vi "Nelson_Whale_Tracker.vi"() -> ()   [LabVIEW 2014]
uses:
  <vilib>/userdefined/High Color/IMAQdx.ctl
  <vilib>/vision/driver/IMAQdx.llb/IMAQdx Attribute Type.ctl
  <vilib>/vision/driver/NI_Vision_Acquisition_Software.lvlib
  <resource>/objmgr/imaqdx.rc
panel:
  in  "Tab Control":enum32{"Whale Tracker", "Diagnostics"}(tab)
  in  "Color Based\nTracking?":bool=TRUE
  out "Image":T1(plugin-control)
  in  "Session In":T2="cam1"
  in  "Image Type":T3=4 items=["Grayscale (U8)", "Grayscale (I16)", "Grayscale (SGL)", "Complex (CSG)", "RGB (U32)", "HSL (U32)", "RGB (U64)", "Grayscale (U16)"]
  out "Whale Position":cluster{"Y":dbl, "X":dbl}
  out "Crosshairs Display":T1(plugin-control)
  in  "Crosshairs Image Type":T3=1 items=["Grayscale (U8)", "Grayscale (I16)", "Grayscale (SGL)", "Complex (CSG)", "RGB (U32)", "HSL (U32)", "RGB (U64)", "Grayscale (U16)"]
  in  "Crosshairs Path":path=path "C:/Users/dnelson1/Desktop/Work/!Classes/Robo I/VISION/2014 Source Images/Crosshairs_Small.bmp"
  out "error out":errorcluster
  out "Attribute Information Array":T5(array[cluster])
  out "Attribute Name":string
  in  "Stop":bool
  out "Running":bool
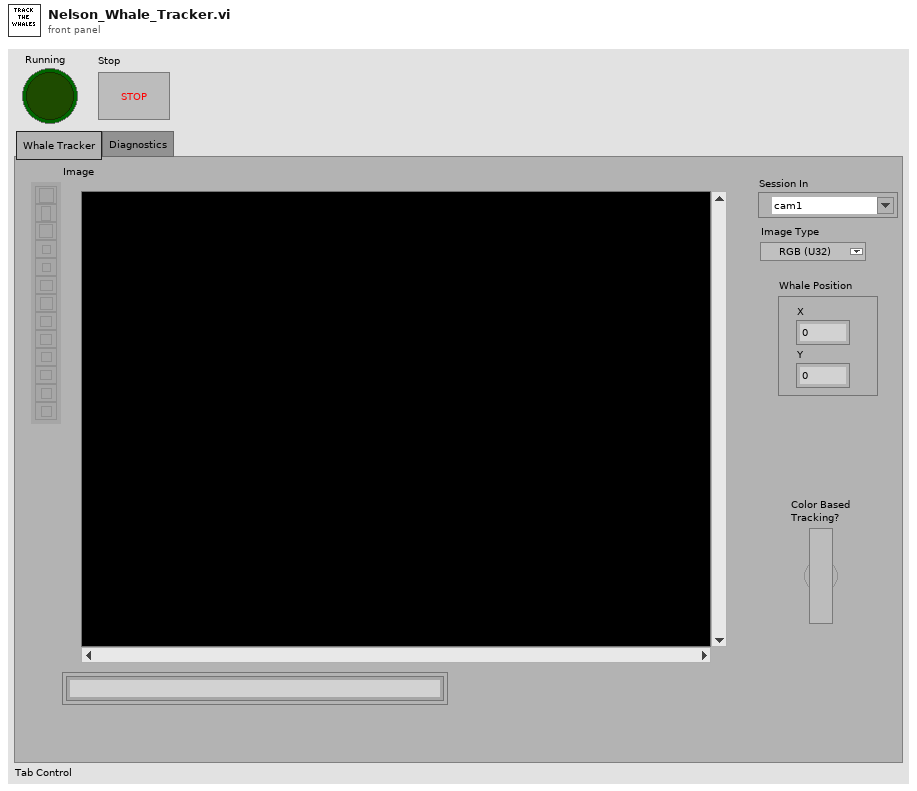
[diagram p1: front panel]
types:
  T1 = typedef "IMAQ Image.ctl" = refnum<image>
  T2 = typedef "IMAQdx.ctl" = refnum<k21>
  T3 = typedef "Image Type" = u32
  T4 = typedef "NI_Vision_Acquisition_Software.lvlib/IMAQdx Attribute Type.ctl" = enum32{"U32", "I64", "DBL", "String", "Enum", "Bool", "Command"}
  T5 = cluster{"Attribute Type":T4, "Readable":bool, "Writable":bool, "Attribute Name":string}[]
  T6 = cluster{"Attribute Type":T4, "Readable":bool, "Writable":bool, "Attribute Name":string}
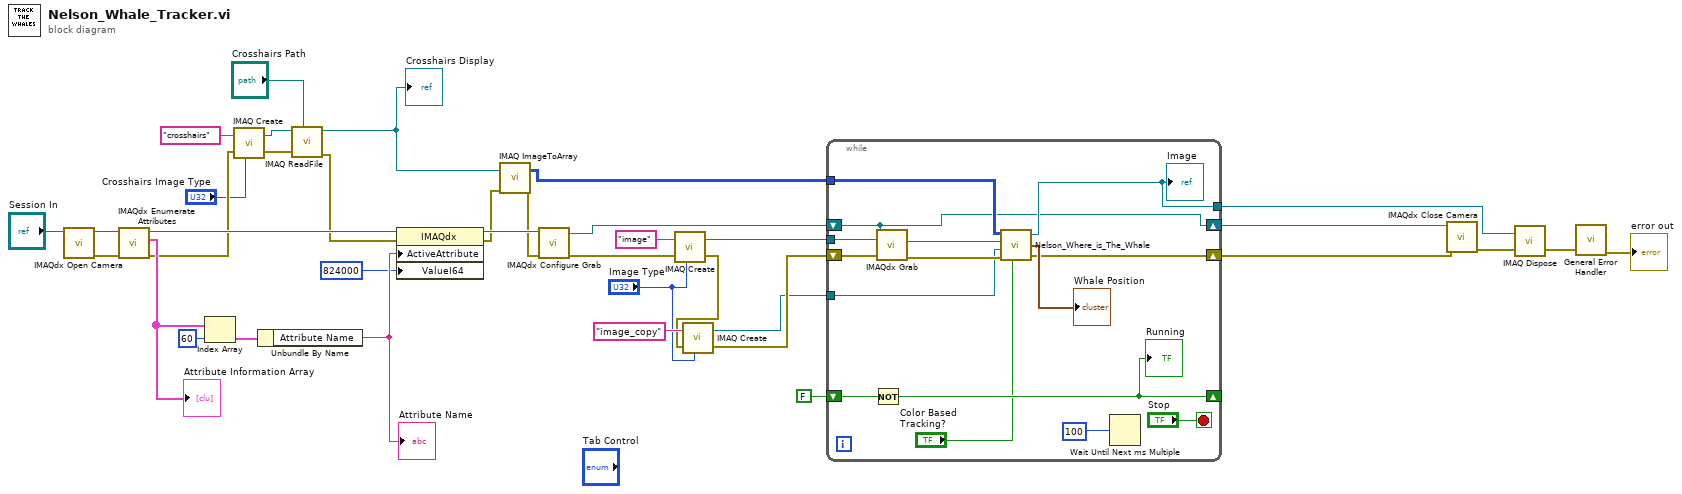
[diagram p0: block diagram]
diagram:
  n1 = call <vilib>:"IMAQdx Open Camera.vi"("Session In"="Session In") -> ("error out"=w35:errorcluster, "Session Out"=w36:T2)  [unwired: 9 in]
  n2 = call <vilib>:"IMAQdx Enumerate Attributes.vi"("error in"=w35, "Session In"=w36) -> ("error out"=w16:errorcluster, "Attribute Information Array"=w32:T5, "Session Out"=w34:T2)  [unwired: 7 in]
  "Attribute Information Array" <- w32
  n3 = Index Array(array=w32, index=60) -> (element=w31:T6)
  n4 = call "IMAQ Create"("Image Name"="crosshairs", "Image Type"="Crosshairs Image Type", "error in (no error)"=w16) -> ("New Image"=w18:T1, "error out"=w17:errorcluster)  [unwired: 2 in]
  n5 = Unbundle By Name(w31) -> ("Attribute Name"=w30:string)
  "Attribute Name" <- w30
  n6 = call "IMAQ ReadFile"("File Path"="Crosshairs Path", "error in (no error)"=w17, "Image"=w18) -> ("error out"=w14:errorcluster, "Image Out"=w10:T1)  [unwired: 4 in, 3 out]
  "Crosshairs Display" <- w10
  n7 = property class="IMAQdx"(reference=w34, error in=w14, "ActiveAttribute"=w30, "ValueI64"=i64 824000) -> (reference out=w28:T2, error out=w2:errorcluster)
  n8 = call "IMAQ ImageToArray"("error in (no error)"=w2, "Image"=w10) -> ("error out"=w1:errorcluster, "Image Pixels (I16)"=w11:i16[][])  [unwired: 2 in, 3 out]
  n9 = call <vilib>:"IMAQdx Configure Grab.vi"("error in"=w1, "Session In"=w28) -> ("error out"=w27:errorcluster, "Session Out"=w24:T2)  [unwired: 8 in]
  n10 = call "IMAQ Create"("Image Name"="image", "Image Type"="Image Type", "error in (no error)"=w27) -> ("New Image"=w25:T1, "error out"=w7:errorcluster)  [unwired: 2 in]
  n11 = call "IMAQ Create"("Image Name"="image_copy", "Image Type"="Image Type", "error in (no error)"=w7) -> ("New Image"=w5:T1, "error out"=w6:errorcluster)  [unwired: 2 in]
  n12 = while {
    shift-right: [w38] -> w21
    shift-left: w24 -> [w38]
    shift-right: [w40] -> w22
    shift-left: w6 -> [w51]
    shift-right: [w48] -> _
    shift-left: FALSE -> [w49]
    tunnel: w11 -> [w42]
    tunnel: w25 -> [w52]
    tunnel: w5 -> [w44]
    tunnel: [w39] -> w4
    stop <- "Stop" stop-if-true
    n13 = Not(x=w49) -> (.not. x?=w48:bool)
    "Running" <- w48
    n14 = call <vilib>:"IMAQdx Grab.vi"("error in"=w51, "Image In"=w52, "Session In"=w38) -> ("error out"=w45:errorcluster, "Image Out"=w43:T1)  [unwired: 5 in, 2 out]
    n15 = call "Nelson_Where_is_The_Whale.vi"("Crosshair Bitmap"=w42, "Image In"=w43, "Image Copy"=w44, "error in"=w45, "Color Based\nTracking?"="Color Based\nTracking?") -> ("Image"=w39:T1, "Whale Position"=→"Whale Position":cluster{"Y":dbl, "X":dbl}, "error out"=w40:errorcluster)
    "Image" <- w39
    n16 = Wait Until Next ms Multiple(millisecond multiple=100) -> ()  [unwired: 1 out]
  }
  n17 = call <vilib>:"IMAQdx Close Camera.vi"("error in"=w22, "Session In"=w21) -> ("error out"=w23:errorcluster)  [unwired: 9 in]
  n18 = call "IMAQ Dispose"("Image"=w4, "error in (no error)"=w23) -> ("error out"=w3:errorcluster)  [unwired: 4 in]
  n19 = call <vilib>:"General Error Handler.vi"("error in (no error)"=w3) -> ("error out"=→"error out":errorcluster)  [unwired: 10 in, 4 out]
